vi "init.vi"(0 "SSR_TTL Low Test in":refnum<class "SSR_TTL Low Test.lvclass">, 5 "ILC":refnum<class "ILC.lvclass">, 7 "ILC Digital Output Test":T1, 9 "Log":refnum<class "ITestLog.lvclass">, 11 "error in (no error)":errorcluster) -> (4 "SSR_TTL Low Test out":refnum<class "SSR_TTL Low Test.lvclass">, 15 "error out":errorcluster)   [LabVIEW 2015, in "SSR_TTL Low Test.lvclass"]
uses:
  SSR_TTL Low Test.lvclass
  Model/TestLog/ITestLog/ITestLog.lvclass
  Typedefs/ILC Digital Output Test.ctl
  Typedefs/Digital Signal Level.ctl
  <userlib>/Common/ILC/ILC/ILC.lvclass
  SSR_TTL Low Test.lvclass/SSR_TTL Low Test.ctl
  Typedefs/ILCBTTypedefs.lvlib
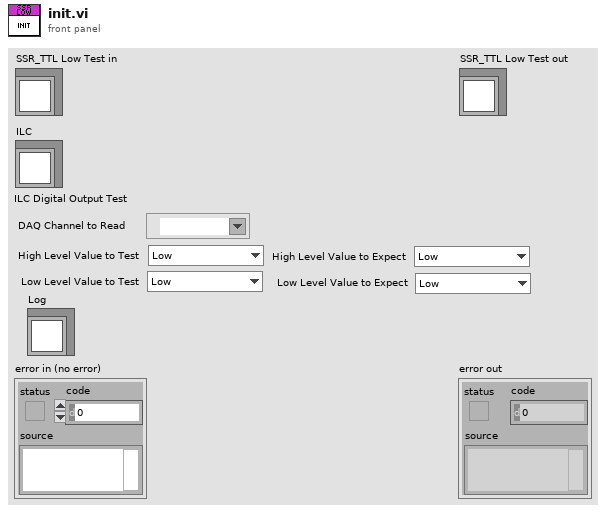
[diagram p1: front panel]
types:
  T1 = typedef "ILCBTTypedefs.lvlib/ILC Digital Output Test.ctl" = cluster{"DAQ Channel to Read":refnum<k21>, "High Level Value to Test":T2, "High Level Value to Expect":T2, "Low Level Value to Test":T2, "Low Level Value to Expect":T2}
  T2 = typedef "ILCBTTypedefs.lvlib/Digital Signal Level.ctl" = enum16{"Low", "High"}
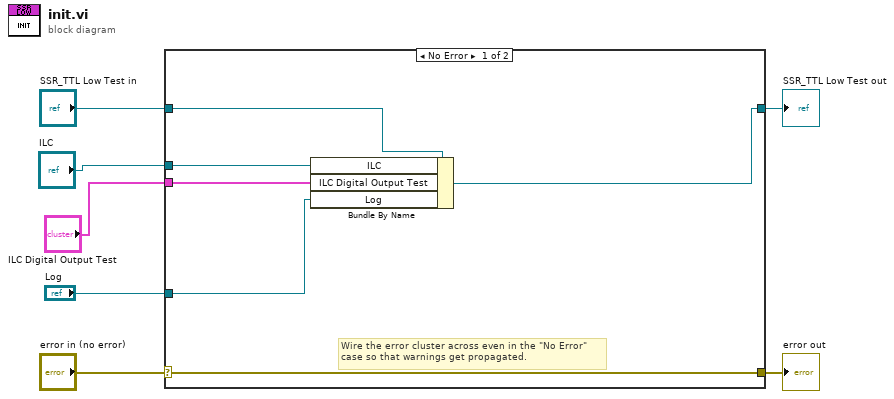
[diagram p0: block diagram]
diagram:
  n1 = case shown="No Error" "error in (no error)" {
    selector: "error in (no error)" -> [w13 w15]
    tunnel: [w13 w15] -> w6
    tunnel: [w8 w14] -> w4
    tunnel: "SSR_TTL Low Test in" -> [w12 w14]
    tunnel: "ILC" -> [w11 _]
    tunnel: "ILC Digital Output Test" -> [w10 _]
    tunnel: "Log" -> [w9 _]
    frame No Error {
      # "Wire the error cluster across even in the \"No Error\"\ncase so that warnings get propagated."
      n2 = Bundle By Name(cluster=w12, "ILC"=w11, "ILC Digital Output Test"=w10, "Log"=w9) -> (w8:refnum<class "SSR_TTL Low Test.lvclass">)
    }
    frame Error {
    }
  }
  "error out" <- w6
  "SSR_TTL Low Test out" <- w4
